vi "GetIrHardwareInfo.vi"(7 "LabVIEW Web Service Request":refnum<class "Web Request.lvclass">) -> ()   [LabVIEW 2017]
uses:
  <vilib>/wsapi/Web Request.lvclass
  <vilib>/addons/InsightCM/MessageBus/Base/controls/KeyValuePair.ctl
  <vilib>/addons/SystemInfoProcess/SystemInfoProcess.lvlib
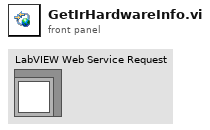
[diagram p1: front panel]
types:
  T1 = typedef "KeyValuePair.ctl" = cluster{"Key":string, "Value":string}
  T2 = typedef "cRIODetectHW.lvlib/SystemHW.ctl" = cluster{"controller":T3, "chassis":T3, "modules":T3[]}
  T3 = typedef "cRIODetectHW.lvlib/cRIO Product Info.ctl" = cluster{"vendorName":string, "productName":string, "serialNumber":string}
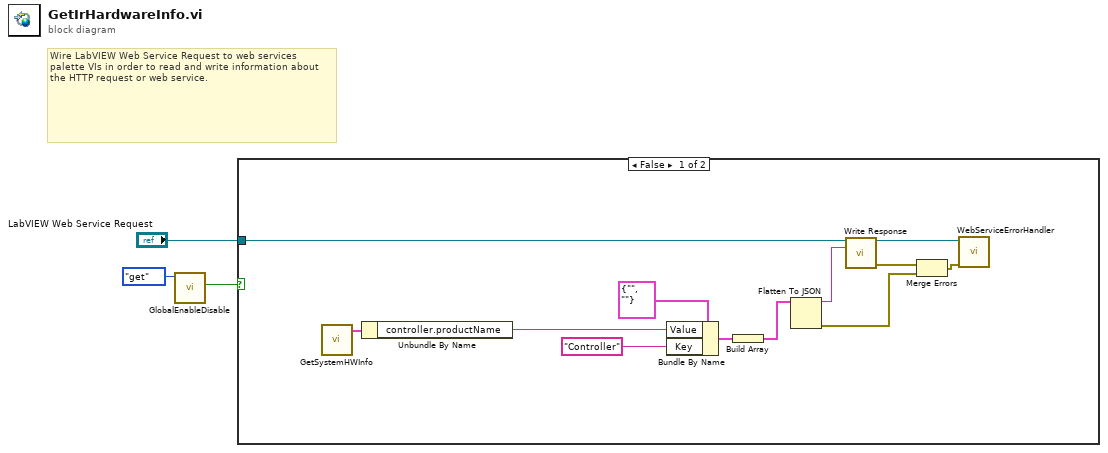
[diagram p0: block diagram]
diagram:
  # "Wire LabVIEW Web Service Request to web services palette VIs in order to read and write information about the HTTP request or web service."
  n1 = call "GlobalEnableDisable.vi"("action"=enum16{"init", "set", "get"}."get") -> ("DisableDeviceWebService"=w2:bool)  [unwired: 10 in]
  n2 = case shown="False" w2 {
    tunnel: "LabVIEW Web Service Request" -> [w10 _]
    frame False {
      n3 = call <vilib>:"GetSystemHWInfo.vi"() -> ("system info"=w7:T2)  [unwired: 9 in, 2 out]
      n4 = Unbundle By Name(w7) -> ("controller.productName"=w6:string)
      n5 = Bundle By Name(cluster=T1 {"Key"="", "Value"=""}, "Value"=w6, "Key"="Controller") -> (w5:T1)
      n6 = Build Array(w5) -> (w4:T1[])
      n7 = Flatten To JSON(anything=w4) -> (JSON string=w15:string, 11:w11:errorcluster)  [unwired: 2 in]
      n8 = call <vilib>:"Write Response.vi"("LabVIEW Web Service Request"=w10, "response string"=w15) -> ("LabVIEW Web Service Request out"=w14:refnum<class "Web Request.lvclass">, "error out"=w13:errorcluster)  [unwired: 12 in]
      n9 = Merge Errors(w13, w11) -> (w12:errorcluster)
      n10 = call "WebServiceErrorHandler.vi"("LabVIEW Web Service Request"=w14, "error in (no error)"=w12) -> ()  [unwired: 12 in, 2 out]
    }
    frame True {
    }
  }
